vi "string_to_float.vi"(8 "error in (no error)":errorcluster, 10 "Float (string)":string) -> (0 "error out":errorcluster, 2 "Float (sgl)":sgl)   [LabVIEW 2018]
doc: "Convert an IC6 response string representing a float into a LabVIEW SGL."
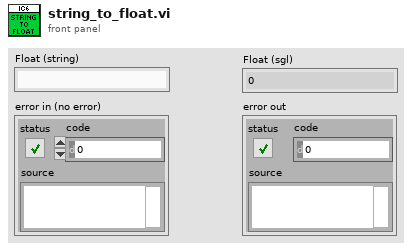
[diagram p1: front panel]
types:
  T1 = enum16{"big-endian, network order", "native, host order", "little-endian"}
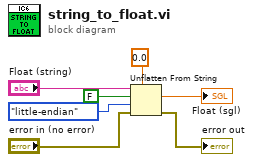
[diagram p0: block diagram]
diagram:
  n1 = Unflatten From String(type=sgl 0.0, binary string="Float (string)", data includes array or string size? (T)=FALSE, byte order (0:big-endian, network order)=T1."little-endian", error in (no error)="error in (no error)") -> (value=→"Float (sgl)":sgl, error out=→"error out":errorcluster)  [unwired: 1 out]
